vi "DDS_Clock.vi"() -> ()   [LabVIEW 2016] (continued)
"f1 [Hz] CH0"=306800000.0}, {"total time[ms]"=38.34999999999996, "f1 [Hz] CH0"=306600000.0}, {"total time[ms]"=38.34999999999996, "f1 [Hz] CH0"=306600000.0}, {"total time[ms]"=38.399999999999956, "f1 [Hz] CH0"=306400000.0}, {"total time[ms]"=38.399999999999956, "f1 [Hz] CH0"=306400000.0}, {"total time[ms]"=38.44999999999995, "f1 [Hz] CH0"=306200000.0}, {"total time[ms]"=38.44999999999995, "f1 [Hz] CH0"=306200000.0}, {"total time[ms]"=38.49999999999995, "f1 [Hz] CH0"=306000000.0}, {"total time[ms]"=38.49999999999995, "f1 [Hz] CH0"=306000000.0}, {"total time[ms]"=38.54999999999995, "f1 [Hz] CH0"=305800000.0}, {"total time[ms]"=38.54999999999995, "f1 [Hz] CH0"=305800000.0}, {"total time[ms]"=38.599999999999945, "f1 [Hz] CH0"=305600000.0}, {"total time[ms]"=38.599999999999945, "f1 [Hz] CH0"=305600000.0}, {"total time[ms]"=38.64999999999994, "f1 [Hz] CH0"=305400000.0}, {"total time[ms]"=38.64999999999994, "f1 [Hz] CH0"=305400000.0}, {"total time[ms]"=38.69999999999994, "f1 [Hz] CH0"=305200000.0}, {"total time[ms]"=38.69999999999994, "f1 [Hz] CH0"=305200000.0}, {"total time[ms]"=38.749999999999936, "f1 [Hz] CH0"=305000000.0}, {"total time[ms]"=38.749999999999936, "f1 [Hz] CH0"=305000000.0}, {"total time[ms]"=38.79999999999993, "f1 [Hz] CH0"=304799999.99999994}, {"total time[ms]"=38.79999999999993, "f1 [Hz] CH0"=304799999.99999994}, {"total time[ms]"=38.84999999999993, "f1 [Hz] CH0"=304600000.0}, {"total time[ms]"=38.84999999999993, "f1 [Hz] CH0"=304600000.0}, {"total time[ms]"=38.89999999999993, "f1 [Hz] CH0"=304400000.0}, {"total time[ms]"=38.89999999999993, "f1 [Hz] CH0"=304400000.0}, {"total time[ms]"=38.949999999999925, "f1 [Hz] CH0"=304200000.0}, {"total time[ms]"=38.949999999999925, "f1 [Hz] CH0"=304200000.0}, {"total time[ms]"=38.99999999999992, "f1 [Hz] CH0"=304000000.0}, {"total time[ms]"=38.99999999999992, "f1 [Hz] CH0"=304000000.0}, {"total time[ms]"=39.04999999999992, "f1 [Hz] CH0"=303800000.0}, {"total time[ms]"=39.04999999999992, "f1 [Hz] CH0"=303800000.0}, {"total time[ms]"=39.099999999999916, "f1 [Hz] CH0"=303600000.0}, {"total time[ms]"=39.099999999999916, "f1 [Hz] CH0"=303600000.0}, {"total time[ms]"=39.14999999999991, "f1 [Hz] CH0"=303399999.99999994}, {"total time[ms]"=39.14999999999991, "f1 [Hz] CH0"=303399999.99999994}, {"total time[ms]"=39.19999999999991, "f1 [Hz] CH0"=303200000.0}, {"total time[ms]"=39.19999999999991, "f1 [Hz] CH0"=303200000.0}, {"total time[ms]"=39.24999999999991, "f1 [Hz] CH0"=303000000.0}, {"total time[ms]"=39.24999999999991, "f1 [Hz] CH0"=303000000.0}, {"total time[ms]"=39.299999999999905, "f1 [Hz] CH0"=302800000.0}, {"total time[ms]"=39.299999999999905, "f1 [Hz] CH0"=302800000.0}, {"total time[ms]"=39.3499999999999, "f1 [Hz] CH0"=302600000.0}, {"total time[ms]"=39.3499999999999, "f1 [Hz] CH0"=302600000.0}, {"total time[ms]"=39.3999999999999, "f1 [Hz] CH0"=302399999.99999994}, {"total time[ms]"=39.3999999999999, "f1 [Hz] CH0"=302399999.99999994}, {"total time[ms]"=39.449999999999896, "f1 [Hz] CH0"=302200000.0}, {"total time[ms]"=39.449999999999896, "f1 [Hz] CH0"=302200000.0}, {"total time[ms]"=39.49999999999989, "f1 [Hz] CH0"=302000000.0}, {"total time[ms]"=39.49999999999989, "f1 [Hz] CH0"=302000000.0}, {"total time[ms]"=39.54999999999989, "f1 [Hz] CH0"=301800000.0}, {"total time[ms]"=39.54999999999989, "f1 [Hz] CH0"=301800000.0}, {"total time[ms]"=39.59999999999989, "f1 [Hz] CH0"=301600000.0}, {"total time[ms]"=39.59999999999989, "f1 [Hz] CH0"=301600000.0}, {"total time[ms]"=39.649999999999885, "f1 [Hz] CH0"=301400000.0}, {"total time[ms]"=39.649999999999885, "f1 [Hz] CH0"=301400000.0}, {"total time[ms]"=39.69999999999988, "f1 [Hz] CH0"=301200000.0}, {"total time[ms]"=39.69999999999988, "f1 [Hz] CH0"=301200000.0}, {"total time[ms]"=39.74999999999988, "f1 [Hz] CH0"=301000000.0}, {"total time[ms]"=39.74999999999988, "f1 [Hz] CH0"=301000000.0}, {"total time[ms]"=39.799999999999876, "f1 [Hz] CH0"=300800000.0}, {"total time[ms]"=39.799999999999876, "f1 [Hz] CH0"=300800000.0}, {"total time[ms]"=39.84999999999987, "f1 [Hz] CH0"=300600000.0}, {"total time[ms]"=39.84999999999987, "f1 [Hz] CH0"=300600000.0}, {"total time[ms]"=39.89999999999987, "f1 [Hz] CH0"=300400000.0}, {"total time[ms]"=39.89999999999987, "f1 [Hz] CH0"=300400000.0}, {"total time[ms]"=39.94999999999987, "f1 [Hz] CH0"=300200000.0}, {"total time[ms]"=39.94999999999987, "f1 [Hz] CH0"=300200000.0}, {"total time[ms]"=39.999999999999865, "f1 [Hz] CH0"=300000000.0}, {"total time[ms]"=39.999999999999865, "f1 [Hz] CH0"=300000000.0}, {"total time[ms]"=40.04999999999986, "f1 [Hz] CH0"=300200000.00000006}, {"total time[ms]"=40.04999999999986, "f1 [Hz] CH0"=300200000.00000006}, {"total time[ms]"=40.09999999999986, "f1 [Hz] CH0"=300400000.0}, {"total time[ms]"=40.09999999999986, "f1 [Hz] CH0"=300400000.0}, {"total time[ms]"=40.14999999999986, "f1 [Hz] CH0"=300600000.0}, {"total time[ms]"=40.14999999999986, "f1 [Hz] CH0"=300600000.0}, {"total time[ms]"=40.199999999999854, "f1 [Hz] CH0"=300800000.0}, {"total time[ms]"=40.199999999999854, "f1 [Hz] CH0"=300800000.0}, {"total time[ms]"=40.24999999999985, "f1 [Hz] CH0"=301000000.0}, {"total time[ms]"=40.24999999999985, "f1 [Hz] CH0"=301000000.0}, {"total time[ms]"=40.29999999999985, "f1 [Hz] CH0"=301200000.0}, {"total time[ms]"=40.29999999999985, "f1 [Hz] CH0"=301200000.0}, {"total time[ms]"=40.349999999999845, "f1 [Hz] CH0"=301400000.0}, {"total time[ms]"=40.349999999999845, "f1 [Hz] CH0"=301400000.0}, {"total time[ms]"=40.39999999999984, "f1 [Hz] CH0"=301600000.00000006}, {"total time[ms]"=40.39999999999984, "f1 [Hz] CH0"=301600000.00000006}, {"total time[ms]"=40.44999999999984, "f1 [Hz] CH0"=301800000.00000006}, {"total time[ms]"=40.44999999999984, "f1 [Hz] CH0"=301800000.00000006}, {"total time[ms]"=40.49999999999984, "f1 [Hz] CH0"=302000000.0}, {"total time[ms]"=40.49999999999984, "f1 [Hz] CH0"=302000000.0}, {"total time[ms]"=40.549999999999834, "f1 [Hz] CH0"=302200000.0}, {"total time[ms]"=40.549999999999834, "f1 [Hz] CH0"=302200000.0}, {"total time[ms]"=40.59999999999983, "f1 [Hz] CH0"=302400000.0}, {"total time[ms]"=40.59999999999983, "f1 [Hz] CH0"=302400000.0}, {"total time[ms]"=40.64999999999983, "f1 [Hz] CH0"=302600000.0}, {"total time[ms]"=40.64999999999983, "f1 [Hz] CH0"=302600000.0}, {"total time[ms]"=40.699999999999825, "f1 [Hz] CH0"=302800000.0}, {"total time[ms]"=40.699999999999825, "f1 [Hz] CH0"=302800000.0}, {"total time[ms]"=40.74999999999982, "f1 [Hz] CH0"=303000000.0}, {"total time[ms]"=40.74999999999982, "f1 [Hz] CH0"=303000000.0}, {"total time[ms]"=40.79999999999982, "f1 [Hz] CH0"=303200000.00000006}, {"total time[ms]"=40.79999999999982, "f1 [Hz] CH0"=303200000.00000006}, {"total time[ms]"=40.84999999999982, "f1 [Hz] CH0"=303400000.0}, {"total time[ms]"=40.84999999999982, "f1 [Hz] CH0"=303400000.0}, {"total time[ms]"=40.899999999999814, "f1 [Hz] CH0"=303600000.0}, {"total time[ms]"=40.899999999999814, "f1 [Hz] CH0"=303600000.0}, {"total time[ms]"=40.94999999999981, "f1 [Hz] CH0"=303800000.0}, {"total time[ms]"=40.94999999999981, "f1 [Hz] CH0"=303800000.0}, {"total time[ms]"=40.99999999999981, "f1 [Hz] CH0"=304000000.0}, {"total time[ms]"=40.99999999999981, "f1 [Hz] CH0"=304000000.0}, {"total time[ms]"=41.049999999999805, "f1 [Hz] CH0"=304200000.0}, {"total time[ms]"=41.049999999999805, "f1 [Hz] CH0"=304200000.0}, {"total time[ms]"=41.0999999999998, "f1 [Hz] CH0"=304400000.0}, {"total time[ms]"=41.0999999999998, "f1 [Hz] CH0"=304400000.0}, {"total time[ms]"=41.1499999999998, "f1 [Hz] CH0"=304600000.00000006}, {"total time[ms]"=41.1499999999998, "f1 [Hz] CH0"=304600000.00000006}, {"total time[ms]"=41.1999999999998, "f1 [Hz] CH0"=304800000.0}, {"total time[ms]"=41.1999999999998, "f1 [Hz] CH0"=304800000.0}, {"total time[ms]"=41.249999999999794, "f1 [Hz] CH0"=305000000.0}, {"total time[ms]"=41.249999999999794, "f1 [Hz] CH0"=305000000.0}, {"total time[ms]"=41.29999999999979, "f1 [Hz] CH0"=305200000.00000006}, {"total time[ms]"=41.29999999999979, "f1 [Hz] CH0"=305200000.00000006}, {"total time[ms]"=41.34999999999979, "f1 [Hz] CH0"=305400000.0}, {"total time[ms]"=41.34999999999979, "f1 [Hz] CH0"=305400000.0}, {"total time[ms]"=41.399999999999785, "f1 [Hz] CH0"=305600000.0}, {"total time[ms]"=41.399999999999785, "f1 [Hz] CH0"=305600000.0}, {"total time[ms]"=41.44999999999978, "f1 [Hz] CH0"=305800000.0}, {"total time[ms]"=41.44999999999978, "f1 [Hz] CH0"=305800000.0}, {"total time[ms]"=41.49999999999978, "f1 [Hz] CH0"=306000000.0}, {"total time[ms]"=41.49999999999978, "f1 [Hz] CH0"=306000000.0}, {"total time[ms]"=41.54999999999978, "f1 [Hz] CH0"=306200000.0}, {"total time[ms]"=41.54999999999978, "f1 [Hz] CH0"=306200000.0}, {"total time[ms]"=41.599999999999774, "f1 [Hz] CH0"=306400000.0}, {"total time[ms]"=41.599999999999774, "f1 [Hz] CH0"=306400000.0}, {"total time[ms]"=41.64999999999977, "f1 [Hz] CH0"=306600000.00000006}, {"total time[ms]"=41.64999999999977, "f1 [Hz] CH0"=306600000.00000006}, {"total time[ms]"=41.69999999999977, "f1 [Hz] CH0"=306800000.00000006}, {"total time[ms]"=41.69999999999977, "f1 [Hz] CH0"=306800000.00000006}, {"total time[ms]"=41.749999999999766, "f1 [Hz] CH0"=307000000.0}, {"total time[ms]"=41.749999999999766, "f1 [Hz] CH0"=307000000.0}, {"total time[ms]"=41.79999999999976, "f1 [Hz] CH0"=307200000.0}, {"total time[ms]"=41.79999999999976, "f1 [Hz] CH0"=307200000.0}, {"total time[ms]"=41.84999999999976, "f1 [Hz] CH0"=307400000.0}, {"total time[ms]"=41.84999999999976, "f1 [Hz] CH0"=307400000.0}, {"total time[ms]"=41.89999999999976, "f1 [Hz] CH0"=307600000.0}, {"total time[ms]"=41.89999999999976, "f1 [Hz] CH0"=307600000.0}, {"total time[ms]"=41.949999999999754, "f1 [Hz] CH0"=307800000.0}, {"total time[ms]"=41.949999999999754, "f1 [Hz] CH0"=307800000.0}, {"total time[ms]"=41.99999999999975, "f1 [Hz] CH0"=308000000.0}, {"total time[ms]"=41.99999999999975, "f1 [Hz] CH0"=308000000.0}, {"total time[ms]"=42.04999999999975, "f1 [Hz] CH0"=308200000.00000006}, {"total time[ms]"=42.04999999999975, "f1 [Hz] CH0"=308200000.00000006}, {"total time[ms]"=42.099999999999746, "f1 [Hz] CH0"=308400000.0}, {"total time[ms]"=42.099999999999746, "f1 [Hz] CH0"=308400000.0}, {"total time[ms]"=42.14999999999974, "f1 [Hz] CH0"=308600000.0}, {"total time[ms]"=42.14999999999974, "f1 [Hz] CH0"=308600000.0}, {"total time[ms]"=42.19999999999974, "f1 [Hz] CH0"=308800000.0}, {"total time[ms]"=42.19999999999974, "f1 [Hz] CH0"=308800000.0}, {"total time[ms]"=42.24999999999974, "f1 [Hz] CH0"=309000000.0}, {"total time[ms]"=42.24999999999974, "f1 [Hz] CH0"=309000000.0}, {"total time[ms]"=42.299999999999734, "f1 [Hz] CH0"=309200000.0}, {"total time[ms]"=42.299999999999734, "f1 [Hz] CH0"=309200000.0}, {"total time[ms]"=42.34999999999973, "f1 [Hz] CH0"=309400000.0}, {"total time[ms]"=42.34999999999973, "f1 [Hz] CH0"=309400000.0}, {"total time[ms]"=42.39999999999973, "f1 [Hz] CH0"=309600000.00000006}, {"total time[ms]"=42.39999999999973, "f1 [Hz] CH0"=309600000.00000006}, {"total time[ms]"=42.449999999999726, "f1 [Hz] CH0"=309800000.0}, {"total time[ms]"=42.449999999999726, "f1 [Hz] CH0"=309800000.0}, {"total time[ms]"=42.49999999999972, "f1 [Hz] CH0"=310000000.0}, {"total time[ms]"=42.49999999999972, "f1 [Hz] CH0"=310000000.0}, {"total time[ms]"=42.54999999999972, "f1 [Hz] CH0"=310200000.00000006}, {"total time[ms]"=42.54999999999972, "f1 [Hz] CH0"=310200000.00000006}, {"total time[ms]"=42.59999999999972, "f1 [Hz] CH0"=310400000.0}, {"total time[ms]"=42.59999999999972, "f1 [Hz] CH0"=310400000.0}, {"total time[ms]"=42.649999999999714, "f1 [Hz] CH0"=310600000.0}, {"total time[ms]"=42.649999999999714, "f1 [Hz] CH0"=310600000.0}, {"total time[ms]"=42.69999999999971, "f1 [Hz] CH0"=310800000.0}, {"total time[ms]"=42.69999999999971, "f1 [Hz] CH0"=310800000.0}, {"total time[ms]"=42.74999999999971, "f1 [Hz] CH0"=311000000.0}, {"total time[ms]"=42.74999999999971, "f1 [Hz] CH0"=311000000.0}, {"total time[ms]"=42.799999999999706, "f1 [Hz] CH0"=311200000.0}, {"total time[ms]"=42.799999999999706, "f1 [Hz] CH0"=311200000.0}, {"total time[ms]"=42.8499999999997, "f1 [Hz] CH0"=311400000.0}, {"total time[ms]"=42.8499999999997, "f1 [Hz] CH0"=311400000.0}, {"total time[ms]"=42.8999999999997, "f1 [Hz] CH0"=311600000.00000006}, {"total time[ms]"=42.8999999999997, "f1 [Hz] CH0"=311600000.00000006}, {"total time[ms]"=42.9499999999997, "f1 [Hz] CH0"=311800000.00000006}, {"total time[ms]"=42.9499999999997, "f1 [Hz] CH0"=311800000.00000006}, {"total time[ms]"=42.999999999999694, "f1 [Hz] CH0"=312000000.0}, {"total time[ms]"=42.999999999999694, "f1 [Hz] CH0"=312000000.0}, {"total time[ms]"=43.04999999999969, "f1 [Hz] CH0"=312200000.0}, {"total time[ms]"=43.04999999999969, "f1 [Hz] CH0"=312200000.0}, {"total time[ms]"=43.09999999999969, "f1 [Hz] CH0"=312400000.0}, {"total time[ms]"=43.09999999999969, "f1 [Hz] CH0"=312400000.0}, {"total time[ms]"=43.149999999999686, "f1 [Hz] CH0"=312600000.0}, {"total time[ms]"=43.149999999999686, "f1 [Hz] CH0"=312600000.0}, {"total time[ms]"=43.19999999999968, "f1 [Hz] CH0"=312800000.0}, {"total time[ms]"=43.19999999999968, "f1 [Hz] CH0"=312800000.0}, {"total time[ms]"=43.24999999999968, "f1 [Hz] CH0"=313000000.0}, {"total time[ms]"=43.24999999999968, "f1 [Hz] CH0"=313000000.0}, {"total time[ms]"=43.29999999999968, "f1 [Hz] CH0"=313200000.00000006}, {"total time[ms]"=43.29999999999968, "f1 [Hz] CH0"=313200000.00000006}, {"total time[ms]"=43.349999999999675, "f1 [Hz] CH0"=313400000.0}, {"total time[ms]"=43.349999999999675, "f1 [Hz] CH0"=313400000.0}, {"total time[ms]"=43.39999999999967, "f1 [Hz] CH0"=313600000.0}, {"total time[ms]"=43.39999999999967, "f1 [Hz] CH0"=313600000.0}, {"total time[ms]"=43.44999999999967, "f1 [Hz] CH0"=313800000.0}, {"total time[ms]"=43.44999999999967, "f1 [Hz] CH0"=313800000.0}, {"total time[ms]"=43.499999999999666, "f1 [Hz] CH0"=314000000.0}, {"total time[ms]"=43.499999999999666, "f1 [Hz] CH0"=314000000.0}, {"total time[ms]"=43.54999999999966, "f1 [Hz] CH0"=314200000.0}, {"total time[ms]"=43.54999999999966, "f1 [Hz] CH0"=314200000.0}, {"total time[ms]"=43.59999999999966, "f1 [Hz] CH0"=314400000.0}, {"total time[ms]"=43.59999999999966, "f1 [Hz] CH0"=314400000.0}, {"total time[ms]"=43.64999999999966, "f1 [Hz] CH0"=314600000.00000006}, {"total time[ms]"=43.64999999999966, "f1 [Hz] CH0"=314600000.00000006}, {"total time[ms]"=43.699999999999655, "f1 [Hz] CH0"=314800000.0}, {"total time[ms]"=43.699999999999655, "f1 [Hz] CH0"=314800000.0}, {"total time[ms]"=43.74999999999965, "f1 [Hz] CH0"=315000000.0}, {"total time[ms]"=43.74999999999965, "f1 [Hz] CH0"=315000000.0}, {"total time[ms]"=43.79999999999965, "f1 [Hz] CH0"=315200000.00000006}, {"total time[ms]"=43.79999999999965, "f1 [Hz] CH0"=315200000.00000006}, {"total time[ms]"=43.849999999999646, "f1 [Hz] CH0"=315400000.0}, {"total time[ms]"=43.849999999999646, "f1 [Hz] CH0"=315400000.0}, {"total time[ms]"=43.89999999999964, "f1 [Hz] CH0"=315600000.0}, {"total time[ms]"=43.89999999999964, "f1 [Hz] CH0"=315600000.0}, {"total time[ms]"=43.94999999999964, "f1 [Hz] CH0"=315800000.0}, {"total time[ms]"=43.94999999999964, "f1 [Hz] CH0"=315800000.0}, {"total time[ms]"=43.99999999999964, "f1 [Hz] CH0"=316000000.0}, {"total time[ms]"=43.99999999999964, "f1 [Hz] CH0"=316000000.0}, {"total time[ms]"=44.049999999999635, "f1 [Hz] CH0"=316200000.0}, {"total time[ms]"=44.049999999999635, "f1 [Hz] CH0"=316200000.0}, {"total time[ms]"=44.09999999999963, "f1 [Hz] CH0"=316400000.0}, {"total time[ms]"=44.09999999999963, "f1 [Hz] CH0"=316400000.0}, {"total time[ms]"=44.14999999999963, "f1 [Hz] CH0"=316600000.00000006}, {"total time[ms]"=44.14999999999963, "f1 [Hz] CH0"=316600000.00000006}, {"total time[ms]"=44.199999999999626, "f1 [Hz] CH0"=316800000.00000006}, {"total time[ms]"=44.199999999999626, "f1 [Hz] CH0"=316800000.00000006}, {"total time[ms]"=44.24999999999962, "f1 [Hz] CH0"=317000000.0}, {"total time[ms]"=44.24999999999962, "f1 [Hz] CH0"=317000000.0}, {"total time[ms]"=44.29999999999962, "f1 [Hz] CH0"=317200000.0}, {"total time[ms]"=44.29999999999962, "f1 [Hz] CH0"=317200000.0}, {"total time[ms]"=44.34999999999962, "f1 [Hz] CH0"=317400000.0}, {"total time[ms]"=44.34999999999962, "f1 [Hz] CH0"=317400000.0}, {"total time[ms]"=44.399999999999615, "f1 [Hz] CH0"=317600000.0}, {"total time[ms]"=44.399999999999615, "f1 [Hz] CH0"=317600000.0}, {"total time[ms]"=44.44999999999961, "f1 [Hz] CH0"=317800000.0}, {"total time[ms]"=44.44999999999961, "f1 [Hz] CH0"=317800000.0}, {"total time[ms]"=44.49999999999961, "f1 [Hz] CH0"=318000000.0}, {"total time[ms]"=44.49999999999961, "f1 [Hz] CH0"=318000000.0}, {"total time[ms]"=44.549999999999606, "f1 [Hz] CH0"=318200000.00000006}, {"total time[ms]"=44.549999999999606, "f1 [Hz] CH0"=318200000.00000006}, {"total time[ms]"=44.5999999999996, "f1 [Hz] CH0"=318400000.0}, {"total time[ms]"=44.5999999999996, "f1 [Hz] CH0"=318400000.0}, {"total time[ms]"=44.6499999999996, "f1 [Hz] CH0"=318600000.0}, {"total time[ms]"=44.6499999999996, "f1 [Hz] CH0"=318600000.0}, {"total time[ms]"=44.6999999999996, "f1 [Hz] CH0"=318800000.0}, {"total time[ms]"=44.6999999999996, "f1 [Hz] CH0"=318800000.0}, {"total time[ms]"=44.749999999999595, "f1 [Hz] CH0"=319000000.0}, {"total time[ms]"=44.749999999999595, "f1 [Hz] CH0"=319000000.0}, {"total time[ms]"=44.79999999999959, "f1 [Hz] CH0"=319200000.0}, {"total time[ms]"=44.79999999999959, "f1 [Hz] CH0"=319200000.0}, {"total time[ms]"=44.84999999999959, "f1 [Hz] CH0"=319400000.0}, {"total time[ms]"=44.84999999999959, "f1 [Hz] CH0"=319400000.0}, {"total time[ms]"=44.89999999999959, "f1 [Hz] CH0"=319600000.00000006}, {"total time[ms]"=44.89999999999959, "f1 [Hz] CH0"=319600000.00000006}, {"total time[ms]"=44.949999999999584, "f1 [Hz] CH0"=319800000.0}, {"total time[ms]"=44.949999999999584, "f1 [Hz] CH0"=319800000.0}, {"total time[ms]"=44.99999999999958, "f1 [Hz] CH0"=320000000.0}, {"total time[ms]"=44.99999999999958, "f1 [Hz] CH0"=320000000.0}, {"total time[ms]"=45.04999999999958, "f1 [Hz] CH0"=319800000.0}, {"total time[ms]"=45.04999999999958, "f1 [Hz] CH0"=319800000.0}, {"total time[ms]"=45.099999999999575, "f1 [Hz] CH0"=319600000.0}, {"total time[ms]"=45.099999999999575, "f1 [Hz] CH0"=319600000.0}, {"total time[ms]"=45.14999999999957, "f1 [Hz] CH0"=319400000.0}, {"total time[ms]"=45.14999999999957, "f1 [Hz] CH0"=319400000.0}, {"total time[ms]"=45.19999999999957, "f1 [Hz] CH0"=319200000.0}, {"total time[ms]"=45.19999999999957, "f1 [Hz] CH0"=319200000.0}, {"total time[ms]"=45.24999999999957, "f1 [Hz] CH0"=319000000.0}, {"total time[ms]"=45.24999999999957, "f1 [Hz] CH0"=319000000.0}, {"total time[ms]"=45.299999999999564, "f1 [Hz] CH0"=318800000.0}, {"total time[ms]"=45.299999999999564, "f1 [Hz] CH0"=318800000.0}, {"total time[ms]"=45.34999999999956, "f1 [Hz] CH0"=318600000.0}, {"total time[ms]"=45.34999999999956, "f1 [Hz] CH0"=318600000.0}, {"total time[ms]"=45.39999999999956, "f1 [Hz] CH0"=318399999.99999994}, {"total time[ms]"=45.39999999999956, "f1 [Hz] CH0"=318399999.99999994}, {"total time[ms]"=45.449999999999555, "f1 [Hz] CH0"=318199999.99999994}, {"total time[ms]"=45.449999999999555, "f1 [Hz] CH0"=318199999.99999994}, {"total time[ms]"=45.49999999999955, "f1 [Hz] CH0"=318000000.0}, {"total time[ms]"=45.49999999999955, "f1 [Hz] CH0"=318000000.0}, {"total time[ms]"=45.54999999999955, "f1 [Hz] CH0"=317800000.0}, {"total time[ms]"=45.54999999999955, "f1 [Hz] CH0"=317800000.0}, {"total time[ms]"=45.59999999999955, "f1 [Hz] CH0"=317600000.0}, {"total time[ms]"=45.59999999999955, "f1 [Hz] CH0"=317600000.0}, {"total time[ms]"=45.649999999999544, "f1 [Hz] CH0"=317400000.0}, {"total time[ms]"=45.649999999999544, "f1 [Hz] CH0"=317400000.0}, {"total time[ms]"=45.69999999999954, "f1 [Hz] CH0"=317200000.0}, {"total time[ms]"=45.69999999999954, "f1 [Hz] CH0"=317200000.0}, {"total time[ms]"=45.74999999999954, "f1 [Hz] CH0"=317000000.0}, {"total time[ms]"=45.74999999999954, "f1 [Hz] CH0"=317000000.0}, {"total time[ms]"=45.799999999999535, "f1 [Hz] CH0"=316799999.99999994}, {"total time[ms]"=45.799999999999535, "f1 [Hz] CH0"=316799999.99999994}, {"total time[ms]"=45.84999999999953, "f1
